vi "WPI_CounterERRIncompatibleMode.vi"() -> (1 "InvalidCounterMode":errorcluster)   [LabVIEW 2017]
doc: "This software is licensed. Open the labview\\readme\\WPI Robotics Library Open Source License.txt file for more information."
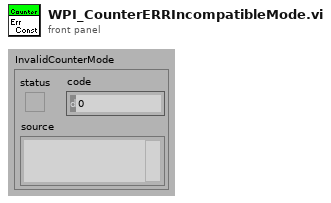
[diagram p1: front panel]
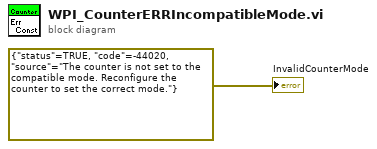
[diagram p0: block diagram]
diagram:
  "InvalidCounterMode" <- errorcluster {"status"=TRUE, "code"=-44020, "source"="The counter is not set to the compatible mode. Reconfigure the counter to set the correct mode."} ("error out 2")
